vi "Get O2 and CLAP MFC Data.vi"(8 "error in":errorcluster, 11 "Serial IO in":refnum<class "Serial IO.lvclass">) -> (0 "error out":errorcluster)   [LabVIEW 2012]
doc: "Get O2 and CLAP MFC data."
uses:
  Reusable/Serial IO/Serial IO.lvclass
  Devices/Alicat/AlicatCommBank/AlicatCommBank.lvclass
  Devices/Alicat/Data/MC/AlicatMCData.lvclass
  Devices/Alicat/Data/VC/AlicatVCData.lvclass
  Devices/Alicat/AlicatCommBank/Set Active Controller on Name.vi
  Devices/Alicat/AlicatCommBank/Get Active Ctl Data.vi
  Reusable/Data/Data.lvclass
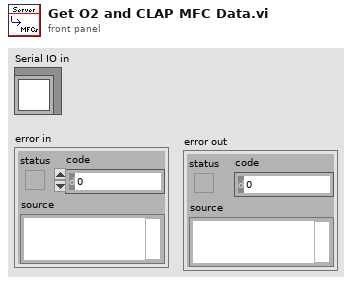
[diagram p1: front panel]
types:
  T1 = cluster{"P":sgl, "T":sgl, "Q":sgl, "Q0":sgl, "Qsp":sgl}
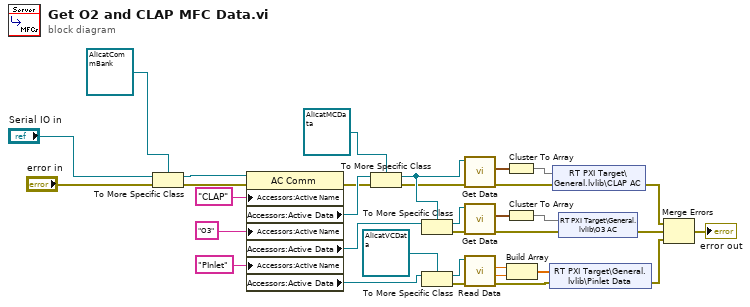
[diagram p0: block diagram]
diagram:
  n1 = To More Specific Class(target class=refnum<class "AlicatCommBank.lvclass"> refnum ("AlicatCommBank in"), reference="Serial IO in", error in="error in") -> (specific class reference=w27:refnum<class "AlicatCommBank.lvclass">, error out=w28:errorcluster)
  n2 = property class="AC Comm"(reference=w27, error in=w28, "Accessors:Active Name"="CLAP" ("Name"), "Accessors:Active Name"="O3" ("Active Name"), "Accessors:Active Name"="PInlet" ("Active Name")) -> (error out=w15:errorcluster, "Accessors:Active Data"=w30:refnum<class "Data.lvclass">, "Accessors:Active Data"=w13:refnum<class "Data.lvclass">, "Accessors:Active Data"=w11:refnum<class "Data.lvclass">)  [unwired: 1 out]
  n3 = To More Specific Class(target class=refnum<class "AlicatMCData.lvclass"> refnum ("AlicatMData in"), reference=w30, error in=w15) -> (specific class reference=w33:refnum<class "AlicatMCData.lvclass">, error out=w32:errorcluster)
  n4 = To More Specific Class(target class=w33, reference=w13) -> (specific class reference=w34:refnum<class "AlicatMCData.lvclass">, error out=w24:errorcluster)  [unwired: 1 in]
  n5 = To More Specific Class(target class=refnum<class "AlicatVCData.lvclass"> refnum ("Alicat.lvlib:AlicatVCData.lvclass"), reference=w11) -> (specific class reference=w21:refnum<class "AlicatVCData.lvclass">, error out=w17:errorcluster)  [unwired: 1 in]
  n6 = call "Get Data.vi"("error in"=w32, "AlicatMData in"=w33) -> ("error out"=w6:errorcluster, "SystemData"=w7:T1)  [unwired: 7 in, 1 out]
  n7 = call "Get Data.vi"("error in"=w24, "AlicatMData in"=w34) -> ("error out"=w5:errorcluster, "SystemData"=w9:T1)  [unwired: 7 in, 1 out]
  n8 = call "Read Data.vi"("error in"=w17, "AlicatVData in"=w21) -> ("error out"=w1:errorcluster, "sp"=w3:sgl, "val"=w4:sgl)  [unwired: 6 in, 1 out]
  n9 = Cluster To Array(cluster=w7) -> (array=w8:sgl[])
  n10 = Cluster To Array(cluster=w9) -> (array=w10:sgl[])
  n11 = Build Array(w4, w3) -> (w2:sgl[])
  n12 = shared-variable "RT PXI Target\\General.lvlib\\Pinlet Data"(w2, error in=w1) -> (error out=w16:errorcluster)
  n13 = shared-variable "RT PXI Target\\General.lvlib\\CLAP AC"(w8, error in=w6) -> (error out=w20:errorcluster)
  n14 = shared-variable "RT PXI Target\\General.lvlib\\O3 AC"(w10, error in=w5) -> (error out=w19:errorcluster)
  n15 = Merge Errors(w20, w19, w16) -> (→"error out":errorcluster)
